vi "Soft_Robot_Model_Conf1.1.vi"() -> ()   [LabVIEW 2015]
uses:
  <vilib>/addons/Control Design/_Stochastic Systems/Stochastic Systems.llb/Stochastic Systems SubVIs/cd_Stochastic State-Space Model.ctl
  <vilib>/addons/Control Design/_Model Construction/Model Typedefs.llb/CD State Space Model (MIMO).ctl
  <vilib>/addons/Control Design/_Model Construction/Model Typedefs.llb/CD General Elements.ctl
  <vilib>/addons/Control Design/_Stochastic Systems/Stochastic Systems.llb/Stochastic Systems SubVIs/cd_Second-Order Statistics Noise Model.ctl
  <vilib>/addons/Control Design/_Stochastic Systems/Stochastic Systems.llb/CD CtoD Stochastic Model.ctl
  <vilib>/Analysis/7linalg.llb/Eigenvalue and Vectors Output Option.ctl
  <vilib>/Platform/TimedLoop/XDataNode/timing_clust.ctl
  <vilib>/Platform/TimedLoop/XDataNode/nitl_modes.ctl
  <vilib>/Platform/TimedLoop/XDataNode/wakeup.ctl
  <vilib>/addons/Control Design/_Stochastic Systems/Stochastic Systems.llb/CD Construct Stochastic Model (Numeric).vi
  <vilib>/Analysis/7linalg.llb/Create Special Real Matrix.vi
  <vilib>/addons/Control Design/_Stochastic Systems/Stochastic Systems.llb/CD Construct Noise Model (Numeric).vi
  <vilib>/addons/Control Design/_State Feedback Control/State Feedback Control.llb/State Feedback Control SubVis/cd_Linear Quadratic Regulator.vi
  <vilib>/Analysis/7linalg.llb/Real Eigenvalues and Vectors.vi
  <vilib>/FPGAPlugInAG/myRIO-1900/niLvFpga_Open_myRIO-1900.vi
  <vilib>/rvi/interface/common/dynamic/niFpgaDynamicAddResources.vi
  <vilib>/Utility/error.llb/Error Cluster From Error Code.vi
  <vilib>/rvi/errors/niLvFpgaAdjustHostInterfaceError.vi
  <vilib>/FPGAPlugInAG/Dynamic/niLvFpga_Close_Dynamic.vi
  <vilib>/Simulation/Estimation/Implementation/NILVSim Discrete Kalman Filter.llb/SIM Disc KF Pred and Corr with Pred Gain with Checking Direct LV.vi
  <vilib>/addons/Control Design/_Implementation/CD State Feedback Controller (Multiple Outputs).vi
  <vilib>/Platform/TimedLoop/XDataNode/XDataNode.xnode
  <vilib>/rvi/interface/nirviOpenFPGA/nirviOpenFPGA.xnode
  FPGA Bitfiles/ACC20115_FPGATarget_CurrentControlle_Dt5vFgOzYtY.lvbitx
  Current Controller.vi
  <vilib>/rvi/interface/nirviReadWriteControl/nirviReadWriteControl.xnode
  <vilib>/rvi/interface/nirviCloseFPGA/nirviCloseFPGA.xnode
  <vilib>/Simulation/Implementation/XNodeFramework/SimXNode/SimX.xnode
  <vilib>/addons/Control Design/_State Feedback Control/NI_CD_State Feedback Control.lvlib
  <vilib>/Analysis/NI_AALPro.lvlib
  <vilib>/Platform/TimedLoop/XDataNode/XDNodeRunTimeDep.lvlib
  <vilib>/rvi/interface/Simulation/niFpgaSimulationCallBeginRW.vi
  <vilib>/addons/Control Design/_Stochastic Systems/NI_CD_Stochastic Systems.lvlib
  <vilib>/addons/Control Design/_State-Space Analysis/NI_CD_State-Space Analysis.lvlib
  NiFpgaLv.dll
  <vilib>/addons/Control Design/_Implementation/NI_CD_Implementation.lvlib
  <vilib>/addons/Control Design/_Model Construction/NI_LinSys_Model Typedefs.lvlib
panel:
  in  "SP":dbl(slide)=666.2985074626865 scale=580.0..720.0
  in  "Tab Control":enum32{"Outputs", "SS Outs", "Inputs"}(tab)
  out "Valve Input Current":dbl(graph)
  out "Status?":bool
  out "Detectable?":bool
  out "Observable?":bool
  out "Controllable?":bool
  out "Stabilizable?":bool
  out "Kinect Fusion":dbl(graph)
  in  "Current (mA)":i32
  out "KF Xhat(k|k)":dbl[][](graph)
  out "Plant Output and KF estimation":dbl[][](graph)=[[689.37, 746.3146706295695]]
  out "KF Predictor Gain L(k)":dbl[][](array[numeric])=[[1.0]] format="%#.6g"
  out "KF Gain M(k)":dbl[][](array[numeric]) format="%#.6g"
  in  "KF R":dbl[](array[slide])=[0.0009999999999999994] scale=0.001..5000.0
  in  "KF Q":dbl[](array[slide])=[208.24576842493772] scale=0.001..5000.0
  in  "Stop":bool
  in  "LQR R":dbl[](array[slide])=[0.14134702368031526] scale=0.001..5000.0
  in  "LQR Matrix (Q)":dbl[](array[slide])=[1000.0000000000007] scale=0.01..1000000.0
  out "LQR Eigenvalues":cdb[](array[numeric]) format="%.5f"
  out "P(k+1|k)":dbl[][](array[numeric])
  out "P(k|k)":dbl[][](array[numeric])
  out "LQR Q Eig Vals":cdb[](array[numeric])
  out "LQR R Eig Val":cdb[](array[numeric])
  out "Optimal LQR Gains":dbl[][](array[numeric])
  out "Stochastic SS Model":T1={"Sampling Time (s)"=0.0, "G"=[], "B"=[[-1.71e-07], [6.47e-07]], "A"=[], "C"=[], "D"=[], "H"=[]} {"H" format="%#.2g"; "D" format="%#.2g"; "C" format="%#.2g"; "A" format="%#.2g"; "B" format="%#.2g"; "G" format="%#.2g"; "Sampling Time (s)" format="%.2f"}
  out "Deterministic SS Model":T2={"properties"={"Model name"="", "Input names"=[], "Output names"=[], "Input Delays"=[], "Output Delays"=[], "Sampling Time"=0.0, "Notes"=""}, "A"=[], "B"=[[-1.706e-07], [6.469e-07]], "C"=[], "D"=[], "StateNames"=[], "Transport Delay"=[]} {"Transport Delay" format="%.2f"; "D" format="%#.2g"; "C" format="%#.2g"; "B" format="%#.2g"; "A" format="%#.2g"; "properties"."Sampling Time" format="%#.6p"; "properties"."Output Delays" format="%.4f"; "properties"."Input Delays" format="%.4f"}
  out "DAC Loop Error":errorcluster
  out "LQR Error":errorcluster
  out "KF Noise Model":T4 {"N" format="%#.2g"; "R" format="%#.2g"; "E{v}" format="%#.2g"; "E{w}" format="%#.2g"; "Q" format="%#.2g"}
  out "FPGA Loop Error":errorcluster
  out "Control Loop Error":errorcluster
  out "KF Model Error":errorcluster
  out "UDP Loop Error":errorcluster
  in  "A":dbl[][](array[numeric])=[[-0.275, -0.05848], [0.3155, 0.05955]] format="%#.5g"
  in  "B":dbl[][](array[numeric])=[[-0.0001629], [8.009e-05]] format="%#.5g"
  in  "C":dbl[][](array[numeric])=[[0.742, 2.316]] format="%#.5g"
  in  "G":dbl[][](array[numeric])=[[0.7998], [2.296]] format="%#.2g"
  in  "xhat(0|-1)":dbl[](array[numeric])=[687.0, 687.0]
  in  "P(0|-1)":dbl[][](array[numeric])=[[1.0, 0.0], [0.0, 1.0]]
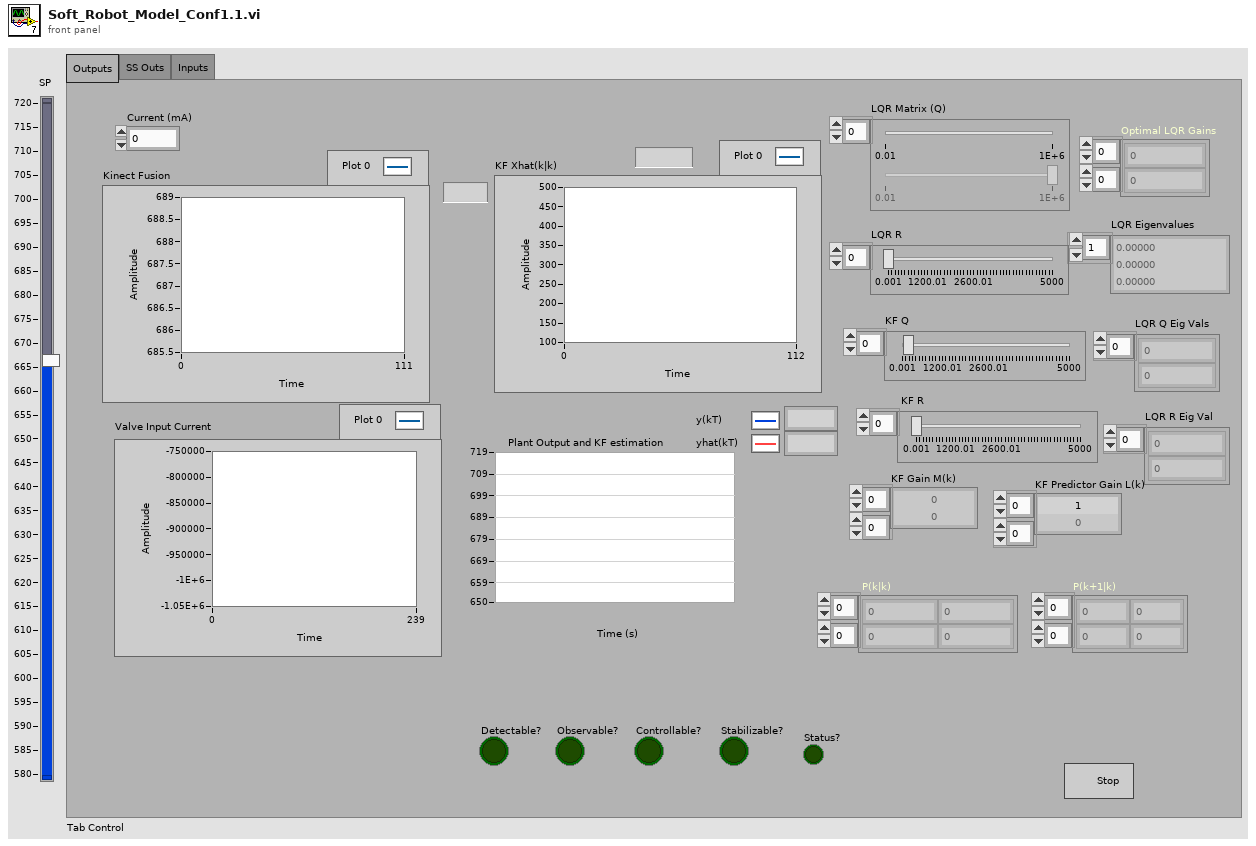
[diagram p1: front panel]
types:
  T1 = typedef "NI_CD_Stochastic Systems.lvlib/cd_Stochastic State-Space Model.ctl" = cluster{"Sampling Time (s)":dbl, "G":dbl[][], "B":dbl[][], "A":dbl[][], "C":dbl[][], "D":dbl[][], "H":dbl[][]}
  T2 = typedef "NI_LinSys_Model Typedefs.lvlib/CD State Space Model (MIMO).ctl" = cluster{"properties":T3, "A":dbl[][], "B":dbl[][], "C":dbl[][], "D":dbl[][], "StateNames":string[], "Transport Delay":dbl[][]}
  T3 = typedef "NI_LinSys_Model Typedefs.lvlib/CD General Elements.ctl" = cluster{"Model name":string, "Input names":string[], "Output names":string[], "Input Delays":dbl[], "Output Delays":dbl[], "Sampling Time":dbl, "Notes":string}
  T4 = typedef "NI_CD_Stochastic Systems.lvlib/cd_Second-Order Statistics Noise Model.ctl" = cluster{"Q":dbl[][], "E{w}":dbl[], "E{v}":dbl[], "R":dbl[][], "N":dbl[][]}
  T5 = typedef "NI_AALPro.lvlib/Eigenvalue and Vectors Output Option.ctl" = i32
  T6 = enum32{"Identity", "Diagonal", "Toepliz", "Vandermonde", "Companion"}
  T7 = typedef "NI_CD_Stochastic Systems.lvlib/CD CtoD Stochastic Model.ctl" = enum16{"Truncation of Taylor Series", "Numerical Integration"}
  T8 = enum16{"state weighting", "output weighting, Dim Q = Ny", "output weighting, Dim Q = Nx"}
  T9 = typedef "NI_Matrix.lvlib/RealMatrix.ctl" = dbl[][]
  T10 = typedef "XDNodeRunTimeDep.lvlib/timing_clust.ctl" = cluster{"Expected End [f-1]":u64, "Actual End [f-1]":u64, "Finished Late? [f-1]":bool, "Expected End [i-1]":u64, "Actual End [i-1]":u64, "Finished Late? [i-1]":bool, "Expected Start [i]":u64, "Actual Start [i]":u64, "Expected Start [f]":u64, "Actual Start [f]":u64, "Source Name":string, "Structure Name":string, "Period":i64, "Deadline":i64, "Offset":i64, "Start":i64, "Priority":i32, "Timeout":i32, "Mode":T11, "Wakeup Reason":T12, "Error":errorcluster, "Source Type":string, "Secondary Source Type":string, "Global End Time":u64, "Global Start Time":u64, "Frame Duration":u64, "Iteration Duration":u64, "Assigned CPU":i32, "I/O Scan Engine Mode":u32}
  T11 = typedef "XDNodeRunTimeDep.lvlib/nitl_modes.ctl" = enum32{"No Change", "Process missed periods, maintain original phase", "Discard missed periods, maintain original phase", "Process missed periods, ignore original phase", "Discard missed periods, ignore original phase"}
  T12 = typedef "XDNodeRunTimeDep.lvlib/wakeup.ctl" = enum32{"Normal", "Aborted", "Asynchronous wakeup", "Timing source error", "Timed loop error", "Timeout"}
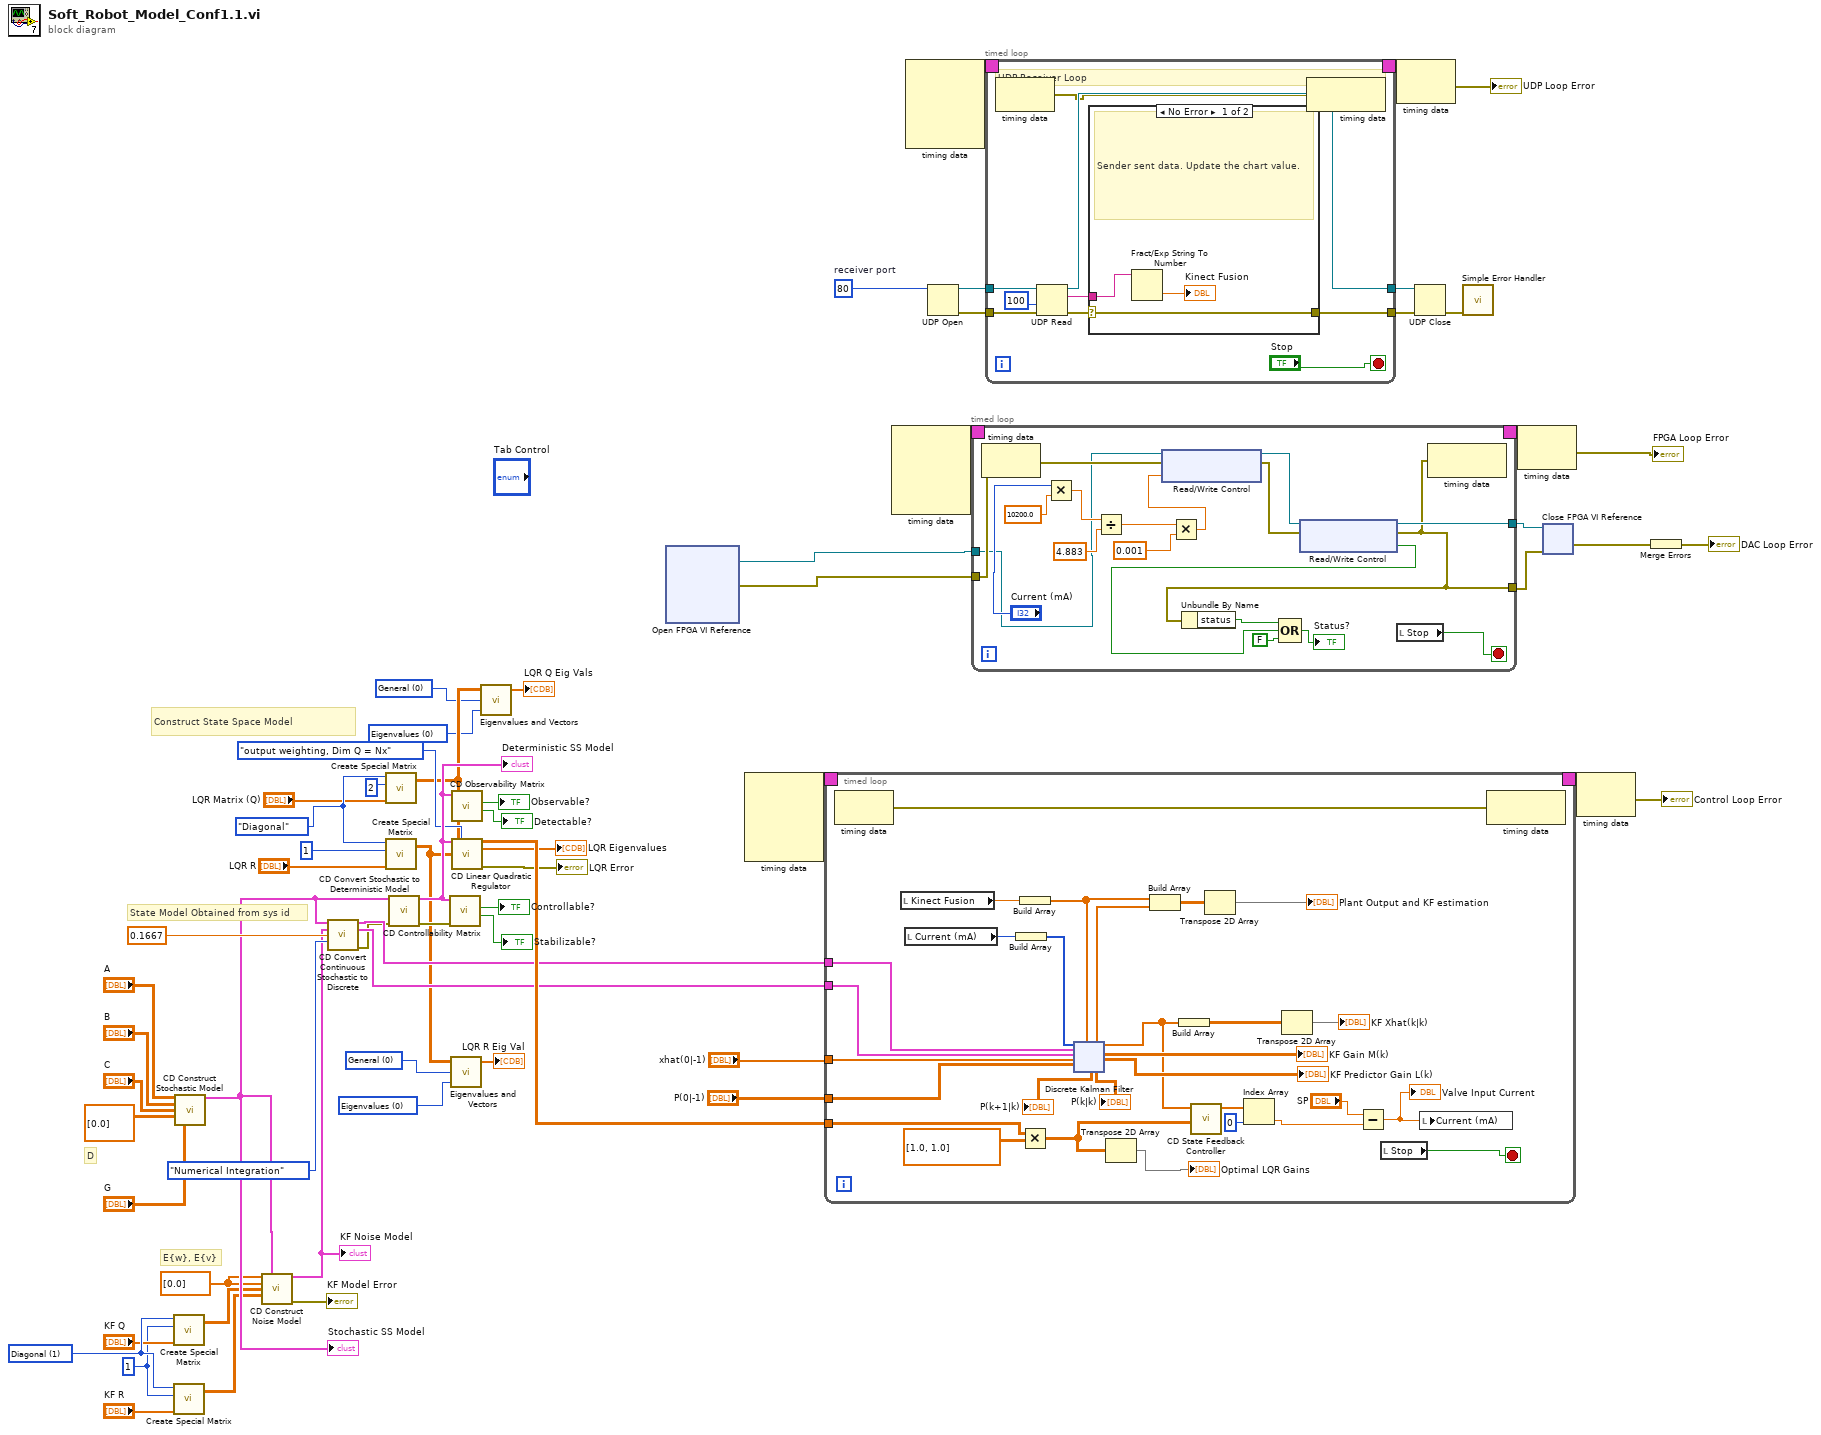
[diagram p0: block diagram]
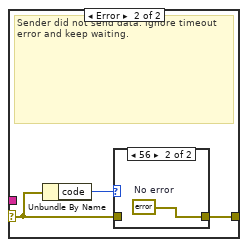
[diagram p2: hidden frame]
diagram:
  w3 = T5 0 items=["Eigenvalues", "Eigenvalues & Vectors"] ("output option")
  w4 = 0 items=["General", "Symmetric"] ("matrix type")
  w6 = T5 0 items=["Eigenvalues", "Eigenvalues & Vectors"] ("output option")
  w7 = 0 items=["General", "Symmetric"] ("matrix type")
  w13 = T6."Diagonal" ("matrix type")
  w14 = 1 ("KF Q/R Size")
  w18 = dbl[] [0.0] ("E{w}")
  w19 = 1 items=["Identity", "Diagonal", "Toeplitz", "Vandermonde", "Companion", "Hankel", "Hadamard", "Wilkinson", "Hilbert", "Inverse Hilbert", "Rosser", "Pascal"] ("matrix type")
  w54 = u16 80  # receiver port
  # "E{w}, E{v}"
  # "D"
  # "State Model Obtained from sys id"
  # "Construct State Space Model"
  n1 = call-poly <vilib>:"Create Special Matrix.vi"("matrix type"=w19, "matrix size"=w14, "Input Vector1"="KF Q") -> ("Special Matrix"=w21:T9)  [unwired: 2 in, 1 out]
  n2 = call-poly <vilib>:"Create Special Matrix.vi"("matrix type"=w19, "matrix size"=w14, "Input Vector1"="KF R") -> ("Special Matrix"=w20:T9)  [unwired: 2 in, 1 out]
  n3 = call-poly <vilib>:"CD Construct Stochastic Model.vi"("A"="A", "B"="B", "C"="C", "D"=dbl[][] [[0.0]], "G"="G") -> ("Stochastic State-Space Model"=w32:T1)  [unwired: 3 in, 7 out]
  "Stochastic SS Model" <- w32
  n4 = call-poly <vilib>:"CD Construct Noise Model.vi"("E{w}"=w18, "Stochastic State-Space Model"=w32, "E{v}"=w18, "Q"=w21, "R"=w20) -> ("Second-Order Statistics Noise Model out"=w33:T4, "error out"=→"KF Model Error":errorcluster)  [unwired: 2 in, 7 out]
  "KF Noise Model" <- w33
  n5 = call <vilib>:"CD Convert Continuous Stochastic to Discrete.vi"("Continuous Stochastic\nState-Space Model"=w32, "Continuous Second-Order\nStatistics Noise Model"=w33, "Sampling Time (s)"=0.1667, "Method"=CD_CtoD_Stochastic_Model."Numerical Integration") -> ("Discrete Stochastic\nState-Space Model"=w43:T1, "Discrete Second-Order\nStatistics Noise Model"=w44:T4, "error out"=w27:errorcluster)  [unwired: 1 in, 8 out]
  n6 = call-poly <vilib>:"Create Special Matrix.vi"("matrix type"=w13, "matrix size"=2, "Input Vector1"="LQR Matrix (Q)") -> ("Special Matrix"=w8:T9)  [unwired: 2 in, 1 out]
  n7 = call-poly <vilib>:"Create Special Matrix.vi"("matrix type"=w13, "matrix size"=1, "Input Vector1"="LQR R") -> ("Special Matrix"=w1:T9)  [unwired: 2 in, 1 out]
  n8 = call <vilib>:"CD Convert Stochastic to Deterministic Model.vi"("Stochastic State-Space Model"=w32, "error in (no error)"=w27) -> ("Deterministic State-Space Model"=w40:T2, "error out"=w26:errorcluster)  [unwired: 12 in]
  "Deterministic SS Model" <- w40
  n9 = call <vilib>:"CD Controllability Matrix.vi"("error in (no error)"=w26, "State-Space Model"=w40) -> ("Is Stabilizable?"=→"Stabilizable?":bool, "Is Controllable?"=→"Controllable?":bool)  [unwired: 6 in, 2 out]
  n10 = call-poly <vilib>:"Eigenvalues and Vectors.vi"("output option"=w3, "matrix type"=w4, "Input Matrix"=w1) -> ("Eigenvalues"=→"LQR R Eig Val":cdb[])  [unwired: 2 out]
  n11 = call <vilib>:"CD Observability Matrix.vi"("State-Space Model"=w40) -> ("Is Detectable?"=→"Detectable?":bool, "Is Observable?"=→"Observable?":bool)  [unwired: 7 in, 2 out]
  n12 = call-poly <vilib>:"CD Linear Quadratic Regulator.vi"("State-Space Model"=w40, "Weighting Type"=T8."output weighting, Dim Q = Nx", "Q"=w8, "R"=w1) -> ("Optimal Gain (K)"=w45:dbl[][], "Eigenvalues"=→"LQR Eigenvalues":cdb[], "error out"=→"LQR Error":errorcluster)  [unwired: 8 in, 1 out]
  n13 = call-poly <vilib>:"Eigenvalues and Vectors.vi"("output option"=w6, "matrix type"=w7, "Input Matrix"=w8) -> ("Eigenvalues"=→"LQR Q Eig Vals":cdb[])  [unwired: 2 out]
  n14 = xnode "Open FPGA VI Reference"() -> ("FPGA VI Reference Out"=w53:refnum<k20>, "error out"=w52:errorcluster)  [unwired: 2 in]
  n15 = node-c288() -> (w47:T10)  [unwired: 4 in]
  n16 = timed-loop {
    timing: w47 -> [_]
    timing-out: [_] -> w46
    tunnel: w45 -> [w71]
    tunnel: w44 -> [w95]
    tunnel: w43 -> [w76]
    tunnel: "xhat(0|-1)" -> [w94]
    tunnel: "P(0|-1)" -> [w93]
    stop <- w73 stop-if-true
    n17 = node-c288() -> (w79:errorcluster)  [unwired: 1 in]
    n18 = local read "Kinect Fusion"() -> (w81:dbl)
    n19 = local read "Current (mA)"() -> (w80:i32)
    n20 = Build Array ("Build Array 5")(w80) -> (w91:i32[])
    n21 = Build Array ("Build Array 3")(w81) -> (w84:dbl[])
    n22 = Multiply(x=w71, y=dbl[][] [[1.0, 1.0]]) -> (x*y=w69:dbl[][])
    n23 = xnode ("Discrete Kalman Filter")("input u(k)"=w91, "Stochastic State-Space Model"=w76, "Second-Order Statistics Noise Model"=w95, "Initial State Estimate xhat(0|-1)"=w94, "Initial Estimation Error Covariance P(0|-1)"=w93, "Output y(k)"=w84) -> ("Prediction Error Covariance P(k+1|k)"=→"P(k+1|k)":dbl[][], "Estimated Output yhat(k)"=w90:dbl[], "Filter Error Covariance P(k|k)"=→"P(k|k)":dbl[][], "Corrected State Estimate xhat(k|k)"=w85:dbl[], "Kalman Filter Gain M(k)"=→"KF Gain M(k)":dbl[][], "Kalman Predictor Gain L(k)"=→"KF Predictor Gain L(k)":dbl[][])  [unwired: 2 in, 2 out]
    n24 = Transpose 2D Array(2D array=w69) -> (transposed array=→"Optimal LQR Gains":dbl[][])
    n25 = Build Array(w84, w90) -> (w89:dbl[][])
    n26 = Build Array ("Build Array 2")(w85) -> (w78:dbl[][])
    n27 = call-poly <vilib>:"CD State Feedback Controller.vi"("Controller Gain"=w69, "States"=w85) -> ("Controller Action"=w92:dbl[])  [unwired: 8 in, 1 out]
    n28 = Transpose 2D Array(2D array=w89) -> (transposed array=→"Plant Output and KF estimation":dbl[][])
    n29 = Index Array(array=w92, index=0) -> (element=w82:dbl)
    n30 = Transpose 2D Array(2D array=w78) -> (transposed array=→"KF Xhat(k|k)":dbl[][])
    n31 = Subtract ("Subtract 2")(x="SP", y=w82) -> (x-y=w77:dbl)
    "Valve Input Current" <- w77
    n32 = local read "Stop"() -> (w73:bool)
    n33 = local write "Current (mA)"(w77) -> ()
    n34 = node-c288(w79) -> ()  [unwired: 1 out]
  }
  n35 = node-c288() -> (w64:T10)  [unwired: 4 in]
  n36 = node-c288() -> (w51:T10)  [unwired: 4 in]
  n37 = UDP Open(11:w54) -> (port=w55:refnum<k16>, 0:w56:errorcluster)  [unwired: 4 in, 1 out]
  n38 = timed-loop {
    tunnel: w52 -> [w120]
    tunnel: [w119] -> w62
    tunnel: [w128] -> w66
    timing: w64 -> [_]
    timing-out: [_] -> w63
    tunnel: w53 -> [w118]
    stop <- w117 stop-if-true
    n39 = node-c288() -> ()  [unwired: 1 in, 1 out]
    n40 = Multiply(x="Current (mA)", y=10200.0) -> (x*y=w123:dbl)
    n41 = Divide(x=w123, y=4.883) -> (x/y=w126:dbl)
    n42 = Multiply(x=w126, y=0.001) -> (x*y=w122:dbl)
    n43 = xnode "Read/Write Control"("FPGA VI Reference In"=w118, "error in"=w120, "DAC Inlet Valve"=w122) -> ("FPGA VI Reference Out"=w134:refnum<k20>, "error out"=w133:errorcluster)
    n44 = xnode "Read/Write Control"("FPGA VI Reference In"=w134, "error in"=w133) -> ("FPGA VI Reference Out"=w128:refnum<k20>, "error out"=w119:errorcluster, "Inlet Overflow?"=w129:bool)
    n45 = Unbundle By Name(w119) -> ("status"=w131:bool)
    n46 = Compound Arithmetic op=OR(w131, w129, FALSE ("value")) -> (→"Status?":bool)
    n47 = local read "Stop"() -> (w117:bool)
    n48 = node-c288(w119) -> ()  [unwired: 1 out]
  }
  n49 = timed-loop {
    tunnel: w55 -> [w147]
    tunnel: [w141] -> w59
    tunnel: w56 -> [w146]
    tunnel: [w142] -> w57
    timing: w51 -> [_]
    timing-out: [_] -> w50
    stop <- "Stop" stop-if-true
    # "UDP Receiver Loop"
    n50 = node-c288() -> (w139:errorcluster)  [unwired: 1 in]
    n51 = UDP Read(connection ID=w147, timeout ms (25000)=100, 8:w146) -> (data out=w144:string, error out=w143:errorcluster, 3:w141:refnum<k16>)  [unwired: 3 out]
    n52 = case shown="No Error" w143 {
      selector: w143 -> [w153 w157]
      tunnel: w144 -> [w155 _]
      tunnel: [w153 w156] -> w142
      frame No Error {
        # "Sender sent data. Update the chart value."
        n53 = Fract/Exp String To Number(string=w155) -> (number=→"Kinect Fusion":dbl)  [unwired: 3 in, 1 out]
      }
      frame Error {
        # "Sender did not send data. Ignore timeout error and keep waiting."
        n54 = Unbundle By Name(w157) -> ("code"=w158:i32)
        n55 = case shown="56" w158 {
          tunnel: w157 -> [w159 _]
          tunnel: [w159 w160] -> w156
          frame Default {
          }
          frame 56 {
            w160 = errorcluster {"status"=FALSE, "code"=0, "source"=""}  # No error
          }
        }
      }
    }
    n56 = node-c288(w139) -> ()  [unwired: 1 out]
  }
  n57 = node-c288(w50) -> (→"UDP Loop Error":errorcluster)
  n58 = UDP Close(connection ID=w59, 8:w57) -> (error out=w58:errorcluster)  [unwired: 1 out]
  n59 = call <vilib>:"Simple Error Handler.vi"("error in (no error)"=w58) -> ()  [unwired: 1 in, 8 out]
  n60 = node-c288(w63) -> (→"FPGA Loop Error":errorcluster)
  n61 = xnode "Close FPGA VI Reference"("FPGA VI Reference In"=w66, "error in"=w62) -> ("error out"=w61:errorcluster)
  n62 = node-c288(w46) -> (→"Control Loop Error":errorcluster)
  n63 = Merge Errors(w61) -> (→"DAC Loop Error":errorcluster)
